vi "macro_AngleStats_AngleMean_CallbackHelp.vi"   [LabVIEW 2019, in "Trajectory_Library.lvlib"]
uses:
  MatBuilder_Create.vi
  Trajectory_Library.lvlib
  AngleStats_AngleMean_CallbackHelp.vi
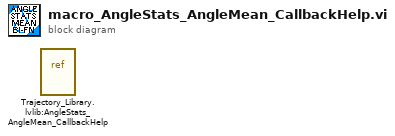
[diagram p0: block diagram]
diagram:
  n1 = vi-ref "Trajectory_Library.lvlib:AngleStats_AngleMean_CallbackHelp.vi"() -> ()  [unwired: 1 out]
